vi "VI Interpreter_String.vi"(8 "error in":errorcluster, 11 "vi name":string) -> (0 "error out":errorcluster, 3 "VI Interpreter out":refnum<class "VI Interpreter.lvclass">)   [LabVIEW 2014, in "Raspberry Pi Compatible Compiler for LabVIEW.lvlib" / "VI Interpreter.lvclass"]
uses:
  VI Interpreter.lvclass
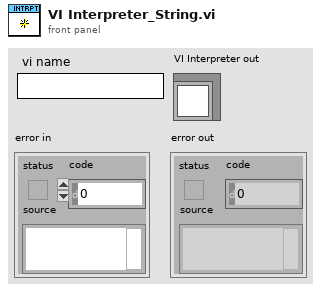
[diagram p1: front panel]
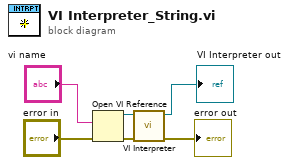
[diagram p0: block diagram]
diagram:
  n1 = Open VI Reference(vi path="vi name", error in (no error)="error in") -> (vi reference=w3:refnum<vi>, error out=w4:errorcluster)  [unwired: 4 in]
  n2 = call "VI Interpreter.vi"("error in"=w4, "vi reference"=w3) -> ("error out"=→"error out":errorcluster, "VI Interpreter out"=→"VI Interpreter out":refnum<class "VI Interpreter.lvclass">)  [unwired: 8 in]
